vi "Determine warnings 2.vi"() -> ()   [LabVIEW 2014]
panel:
  out "Warning?":bool
  out "Warning Text":string
  in  "Max Temp":dbl
  in  "Min Temp":dbl
  in  "Current Temp":dbl
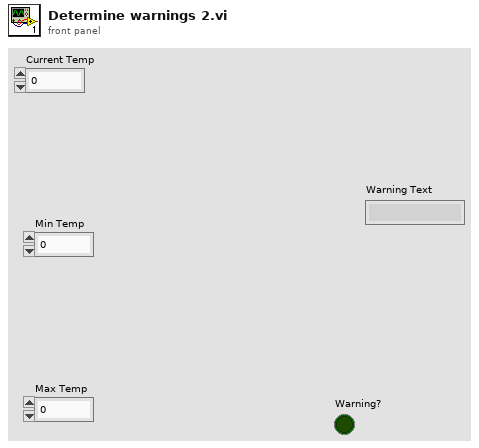
[diagram p1: front panel]
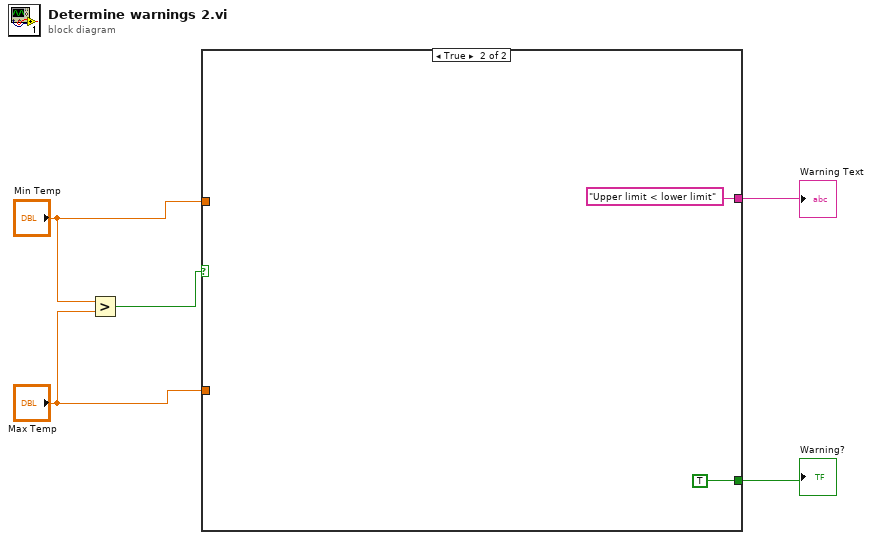
[diagram p0: block diagram]
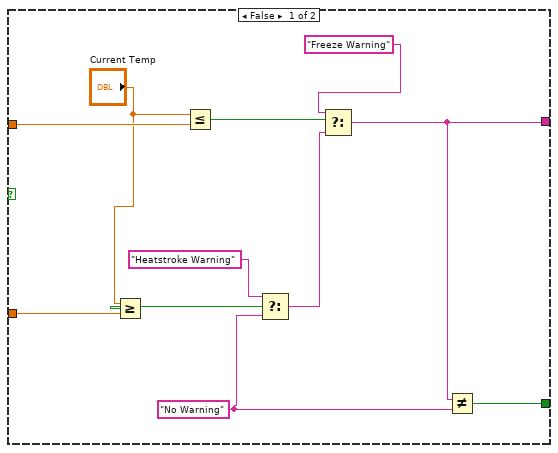
[diagram p2: hidden frame]
diagram:
  n1 = Greater?(x="Min Temp", y="Max Temp") -> (0:w1:bool)
  n2 = case shown="True" w1 {
    tunnel: "Min Temp" -> [w16 _]
    tunnel: "Max Temp" -> [w15 _]
    tunnel: [w7 "Upper limit < lower limit"] -> w5
    tunnel: [w6 TRUE ("Warning?")] -> w4
    frame False {
      w8 = "No Warning"
      n3 = Greater Or Equal?(x="Current Temp", y=w15) -> (x >= y?=w13:bool)
      n4 = Less Or Equal?(x="Current Temp", y=w16) -> (x <= y?=w11:bool)
      n5 = Select(t="Heatstroke Warning", s=w13, f=w8) -> (s? t:f=w9:string)
      n6 = Select(t="Freeze Warning", s=w11, f=w9) -> (s? t:f=w7:string)
      n7 = Not Equal?(x=w7, y=w8) -> (x != y?=w6:bool)
    }
    frame True {
    }
  }
  "Warning Text" <- w5
  "Warning?" <- w4
